vi "testK3390.vi"() -> ()   [LabVIEW 2009, in "run.lvlib"]
uses:
  run.lvlib
  <instrlib>/Keithley 3390/Public/Configure/Low Level/Configure Voltage (Amplitude).vi
  <instrlib>/Keithley 3390/Keithley 3390.lvlib
  <instrlib>/Keithley 3390/Public/Configure/Configure Waveform (Sine).vi
panel:
  in  "DC Offset (0.00 V)":dbl
  in  "Amplitude (1.0 Vpp)":dbl=1.0 format="%.3g"
  in  "Frequency (kHz)":dbl=24.0 format="%_5g"
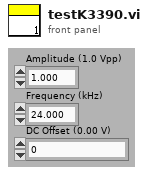
[diagram p1: front panel]
types:
  T1 = enum16{"Sine", "Square", "Ramp", "Pulse", "Noise", "DC", "Arbitrary"}
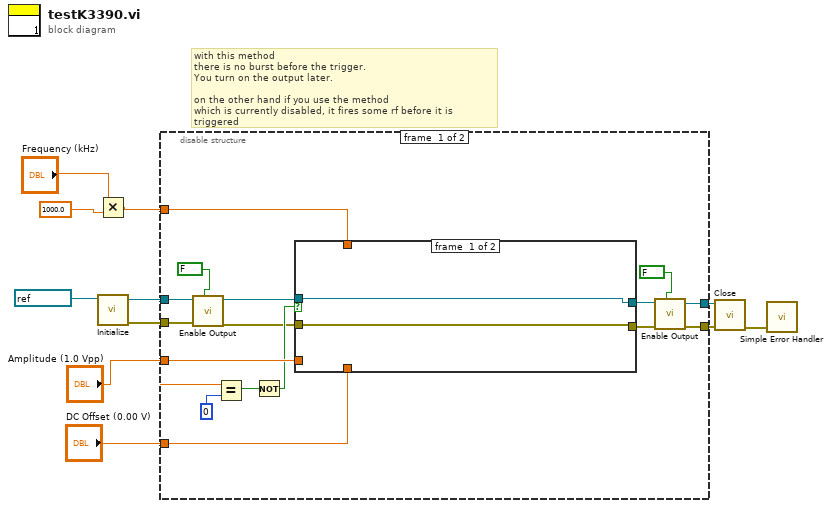
[diagram p0: block diagram]
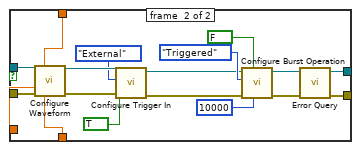
[diagram p2: hidden frame]
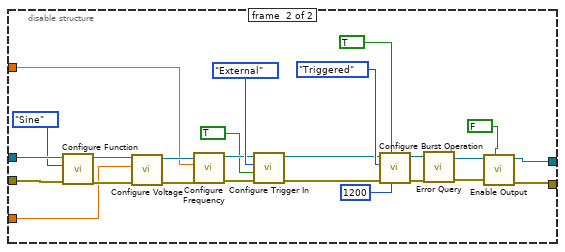
[diagram p3: hidden frame]
diagram:
  # "with this method\nthere is no burst before the trigger.\nYou turn on the output later.\n\non the other hand if you use the method\nwhich is currently disabled, it fires some rf before it is triggered"
  n1 = Multiply(x="Frequency (kHz)", y=1000.0) -> (x*y=w1:dbl)
  n2 = call <instrlib>:"Initialize.vi"("VISA resource name"=refnum<visa-resource-name> "k3390") -> ("error out"=w4:errorcluster, "VISA resource name out"=w5:refnum<visa-resource-name>)  [unwired: 9 in]
  n3 = disable-structure shown="Enabled" {
    disable-tunnel: "DC Offset (0.00 V)" -> [w27 _]
    disable-tunnel: [w26 w49] -> w9
    disable-tunnel: [w25 w50] -> w8
    disable-tunnel: "Amplitude (1.0 Vpp)" -> [w24 w67]
    disable-tunnel: w5 -> [w23 w72]
    disable-tunnel: w4 -> [w22 w71]
    disable-tunnel: w1 -> [w21 w65]
    frame #0 {
      n4 = call <instrlib>:"Enable Output.vi"("Enable Output (T: Enable)"=FALSE, "error in (no error)"=w22, "VISA resource name"=w23) -> ("error out"=w13:errorcluster, "VISA resource name out"=w12:refnum<visa-resource-name>)  [unwired: 7 in]
      n5 = Equal?(x=w24, y=0) -> (x = y?=w17:bool)
      n6 = Not(x=w17) -> (.not. x?=w16:bool)
      n7 = case shown="True" w16 {
        tunnel: w12 -> [w29 w47]
        tunnel: w13 -> [w28 w46]
        tunnel: w21 -> [_ w45]
        tunnel: w27 -> [_ w44]
        tunnel: [w29 w33] -> w20
        tunnel: [w28 w32] -> w19
        tunnel: w24 -> [_ w31]
        frame #0 {
        }
        frame #1 {
          n8 = call-poly <instrlib>:"Configure Waveform.vi"("VISA resource name"=w47, "Frequency (1000 Hz)"=w45, "Amplitude (1.0 Vpp)"=w31, "error in (no error)"=w46, "DC Offset (0.00 V)"=w44) -> ("VISA resource name out"=w39:refnum<visa-resource-name>, "error out"=w40:errorcluster)  [unwired: 9 in]
          n9 = call <instrlib>:"Configure Trigger In.vi"("error in (no error)"=w40, "External Trigger Slope (T: Positive)"=TRUE, "Trigger Source (0:Immediate)"=enum16{"Immediate", "External", "Bus"}."External", "VISA resource name"=w39) -> ("error out"=w36:errorcluster, "VISA resource name out"=w37:refnum<visa-resource-name>)  [unwired: 6 in]
          n10 = call <instrlib>:"Configure Burst Operation.vi"("Burst Count (1)"=10000, "Enable Burst Operation (Enable)"=FALSE, "error in (no error)"=w36, "Burst Mode (Triggered)"=enum16{"Triggered", "Gated"}."Triggered", "VISA resource name"=w37) -> ("error out"=w34:errorcluster, "VISA resource name out"=w35:refnum<visa-resource-name>)  [unwired: 5 in]
          n11 = call <instrlib>:"Error Query.vi"("error in (no error)"=w34, "VISA resource name"=w35) -> ("error out"=w32:errorcluster, "VISA resource name out"=w33:refnum<visa-resource-name>)  [unwired: 6 in, 2 out]
        }
      }
      n12 = call <instrlib>:"Enable Output.vi"("Enable Output (T: Enable)"=FALSE, "error in (no error)"=w19, "VISA resource name"=w20) -> ("error out"=w26:errorcluster, "VISA resource name out"=w25:refnum<visa-resource-name>)  [unwired: 7 in]
    }
    frame #1 {
      n13 = call <instrlib>:"Configure Function.vi"("error in (no error)"=w71, "Function (Sine)"=T1."Sine", "VISA resource name"=w72) -> ("error out"=w68:errorcluster, "VISA resource name out"=w69:refnum<visa-resource-name>)  [unwired: 7 in]
      n14 = call-poly <instrlib>:"Configure Voltage.vi"("error in (no error)"=w68, "Amplitude (1.00 Vpp)"=w67, "VISA resource name"=w69) -> ("error out"=w64:errorcluster, "VISA resource name out"=w66:refnum<visa-resource-name>)  [unwired: 7 in]
      n15 = call <instrlib>:"Configure Frequency.vi"("error in (no error)"=w64, "Frequency (1000 Hz)"=w65, "VISA resource name"=w66) -> ("error out"=w52:errorcluster, "VISA resource name out"=w53:refnum<visa-resource-name>)  [unwired: 7 in]
      n16 = call <instrlib>:"Configure Trigger In.vi"("error in (no error)"=w52, "External Trigger Slope (T: Positive)"=TRUE, "Trigger Source (0:Immediate)"=enum16{"Immediate", "External", "Bus"}."External", "VISA resource name"=w53) -> ("error out"=w58:errorcluster, "VISA resource name out"=w59:refnum<visa-resource-name>)  [unwired: 6 in]
      n17 = call <instrlib>:"Configure Burst Operation.vi"("Burst Count (1)"=1200, "Enable Burst Operation (Enable)"=TRUE, "error in (no error)"=w58, "Burst Mode (Triggered)"=enum16{"Triggered", "Gated"}."Triggered", "VISA resource name"=w59) -> ("error out"=w56:errorcluster, "VISA resource name out"=w57:refnum<visa-resource-name>)  [unwired: 5 in]
      n18 = call <instrlib>:"Error Query.vi"("error in (no error)"=w56, "VISA resource name"=w57) -> ("error out"=w55:errorcluster, "VISA resource name out"=w54:refnum<visa-resource-name>)  [unwired: 6 in, 2 out]
      n19 = call <instrlib>:"Enable Output.vi"("Enable Output (T: Enable)"=FALSE, "error in (no error)"=w55, "VISA resource name"=w54) -> ("error out"=w49:errorcluster, "VISA resource name out"=w50:refnum<visa-resource-name>)  [unwired: 7 in]
    }
  }
  n20 = call <instrlib>:"Close.vi"("error in (no error)"=w9, "VISA resource name"=w8) -> ("error out"=w7:errorcluster)  [unwired: 9 in]
  n21 = call <vilib>:"Simple Error Handler.vi"("error in (no error)"=w7) -> ()  [unwired: 4 in, 5 out]
